vi "mirror trans dat.vi"() -> ()   [LabVIEW 2016]
panel:
  out "Flattened Transconductance 2":dbl[][](graph)
  in  "Flattened Transconductance":dbl[][](graph)
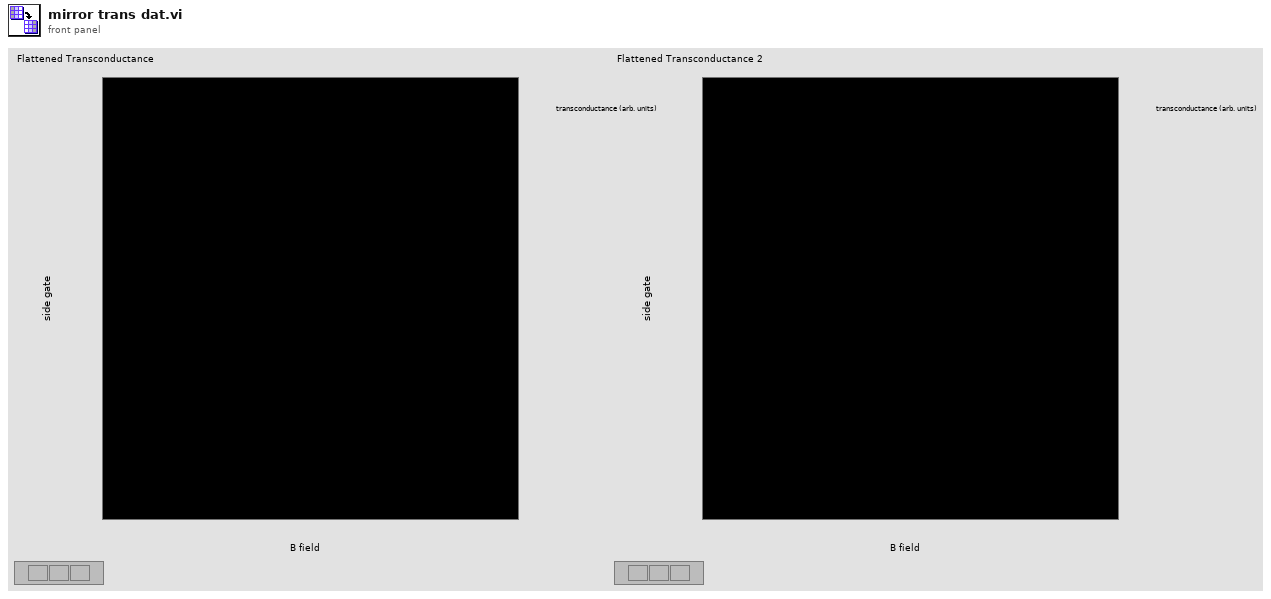
[diagram p1: front panel]
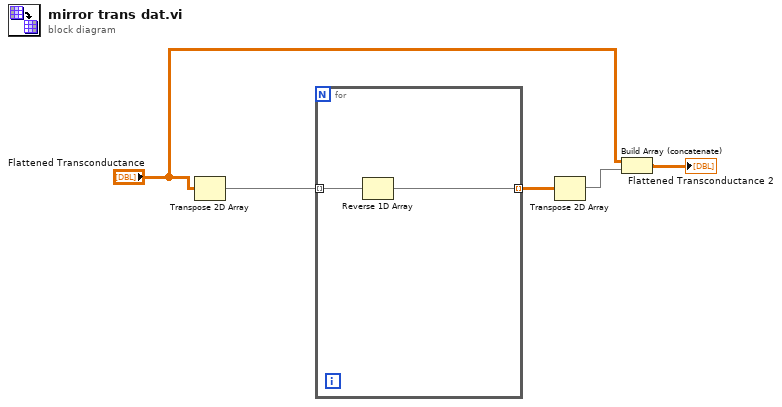
[diagram p0: block diagram]
diagram:
  n1 = Transpose 2D Array(2D array="Flattened Transconductance") -> (transposed array=w5:dbl[][])
  n2 = for {
    tunnel: w5 -> [w7] mode=indexing
    tunnel: [w6] -> w4 mode=indexing
    n3 = Reverse 1D Array(array=w7) -> (reversed array=w6:dbl[])
  }
  n4 = Transpose 2D Array(2D array=w4) -> (transposed array=w2:dbl[][])
  n5 = Build Array (concatenate)("Flattened Transconductance", w2) -> (→"Flattened Transconductance 2":dbl[][])
